vi "VSG_SET-GET_AMPL_3.00.vi"(4 "delay after set (s)":dbl caption="Delay Time (s)", 6 "Get Power Only (T)":bool, 8 "error in":errorcluster {"code" format="%.0x"}, 9 "Set Power (num)":dbl=-25.0, 10 "Offset (dB)":dbl, 11 "Session In":refnum<visa-resource-name>="GPIB0::18::INSTR") -> (0 "error out":errorcluster {"code" format="%.0x"}, 1 "Get Power":dbl=-25.0, 3 "Session Out":refnum<visa-resource-name>="GPIB0::18::INSTR")   [LabVIEW 2018]
doc: "Set/Get the ESG RF Amplitude in current units.\n\nV2.00 Added error query to avoid overdriving.Also will shut power off if too high."
panel:
  in  "Timeout":u32=3000
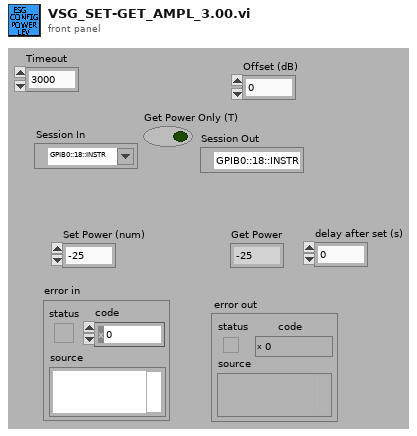
[diagram p1: front panel]
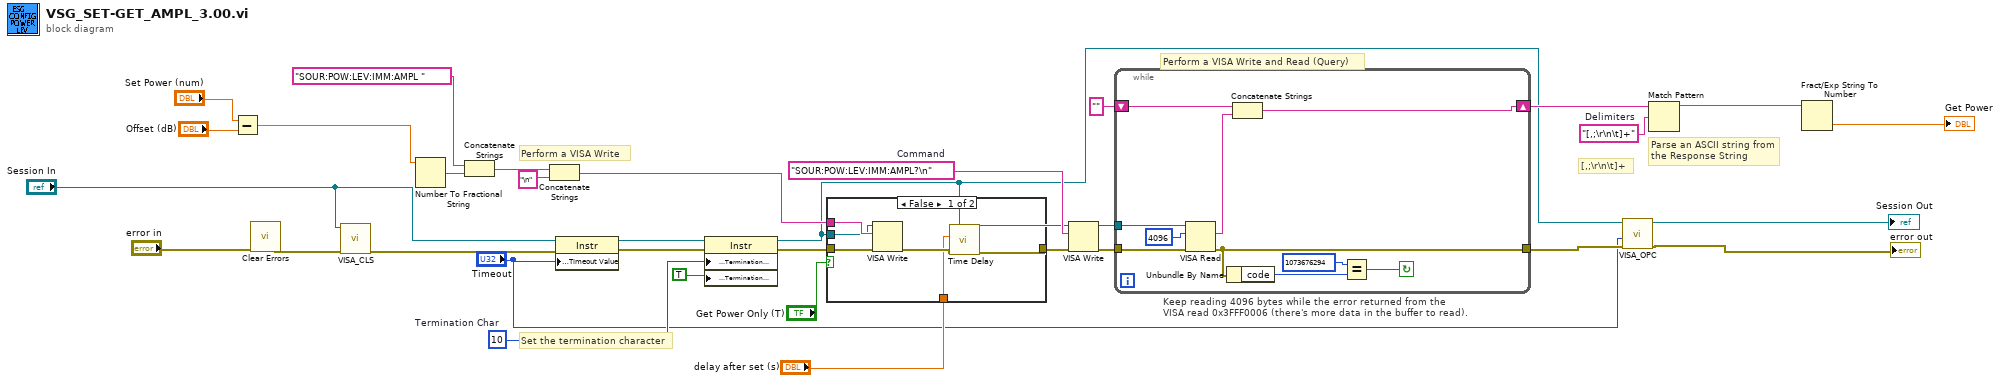
[diagram p0: block diagram]
diagram:
  w16 = "[,;\r\n\t]+"  # Delimiters
  w17 = "SOUR:POW:LEV:IMM:AMPL?\n"  # Command
  w29 = u8 10  # Termination Char
  # "[,;\\r\\n\\t]+"
  # "Parse an ASCII string from the Response String"
  # "Perform a VISA Write and Read (Query)"
  # "Keep reading 4096 bytes while the error returned from the\nVISA read 0x3FFF0006 (there's more data in the buffer to read)."
  # "Perform a VISA Write"
  # "Set the termination character"
  n1 = Subtract(x="Set Power (num)", y="Offset (dB)") -> (x-y=w6:dbl)
  n2 = call <vilib>:"Clear Errors.vi"("error in (no error)"="error in") -> ("error out"=w10:errorcluster)  [unwired: 5 in, 1 out]
  n3 = call "VISA_CLS.vi"("error in"=w10, "Session In"="Session In") -> ("error out"=w9:errorcluster)  [unwired: 8 in, 1 out]
  n4 = Number To Fractional String(number=w6) -> (F-format string=w15:string)  [unwired: 3 in]
  n5 = Concatenate Strings("SOUR:POW:LEV:IMM:AMPL " ("staticText"), w15) -> (w27:string)
  n6 = Concatenate Strings(w27, "\n" ("StaticText")) -> (w24:string)
  n7 = property class="Instr"(reference="Session In", error in=w9, "General Settings:Timeout Value"="Timeout") -> (reference out=w32:refnum<visa-resource-name>, error out=w31:errorcluster)
  n8 = property class="Instr"(reference=w32, error in=w31, "Message Based Settings:Termination Character"=w29, "Message Based Settings:Termination Character Enable"=TRUE ("enable")) -> (reference out=w14:refnum<visa-resource-name>, error out=w30:errorcluster)
  n9 = case shown="False" "Get Power Only (T)" {
    tunnel: w30 -> [w39 w40]
    tunnel: [w36 w40] -> w25
    tunnel: w24 -> [w38 _]
    tunnel: w14 -> [w37 _]
    tunnel: "delay after set (s)" -> [w34 _]
    frame False {
      n10 = VISA Write(VISA resource name=w37, write buffer=w38, error in (no error)=w39) -> (error out=w35:errorcluster)  [unwired: 2 out]
      n11 = call "Time Delay"("error in (no error)"=w35, "Delay Time (s)"=w34) -> ("error out"=w36:errorcluster)  [unwired: 9 in]
    }
    frame True {
    }
  }
  n12 = VISA Write(VISA resource name=w14, write buffer=w17, error in (no error)=w25) -> (VISA resource name out=w22:refnum<visa-resource-name>, error out=w20:errorcluster)  [unwired: 1 out]
  n13 = while {
    tunnel: w22 -> [w47]
    shift-right: [w41] -> w21
    shift-left: "" -> [w46]
    tunnel: w20 -> [w44]
    tunnel: [w43] -> w19
    stop <- w42 continue-if-true
    n14 = VISA Read(VISA resource name=w47, byte count=u32 4096 ("byte count (0)"), error in (no error)=w44) -> (read buffer=w45:string, error out=w43:errorcluster)  [unwired: 2 out]
    n15 = Unbundle By Name(w43) -> ("code"=w49:i32)
    n16 = Concatenate Strings(w46, w45) -> (w41:string)
    n17 = Equal?(x=1073676294, y=w49) -> (x = y?=w42:bool)
  }
  n18 = call "VISA_OPC.vi"("error in"=w19, "Timeout"="Timeout", "Session In"=w14) -> ("error out"=→"error out":errorcluster, "Session Out"=→"Session Out":refnum<visa-resource-name>)  [unwired: 6 in, 1 out]
  n19 = Match Pattern(string=w21, regular expression=w16) -> (before substring=w12:string)  [unwired: 1 in, 3 out]
  n20 = Fract/Exp String To Number(string=w12) -> (number=→"Get Power":dbl)  [unwired: 3 in, 1 out]
